vi "gui-demo.vi"() -> ()   [LabVIEW 2017]
uses:
  event-message-data.ctl
  list-commands-names.ctl
panel:
  in  "Array - String":string[](array[string])
  in  "create":bool
  in  "Instruction Tamplate":T1[](array[typedef])
  out "value":T2
  in  "stop":bool
  out "Instruction":string
  in  "initial preset":T3={"command-stack"=["label1:WAIT_SECONDS,2", "LIBX,demo-testflow.vi,WAIT", "JUMPCNT,label1,1", "FINISH"], "stack-config"=""}
  out "Instruction":string
  out "WAIT_SECONDS":T4
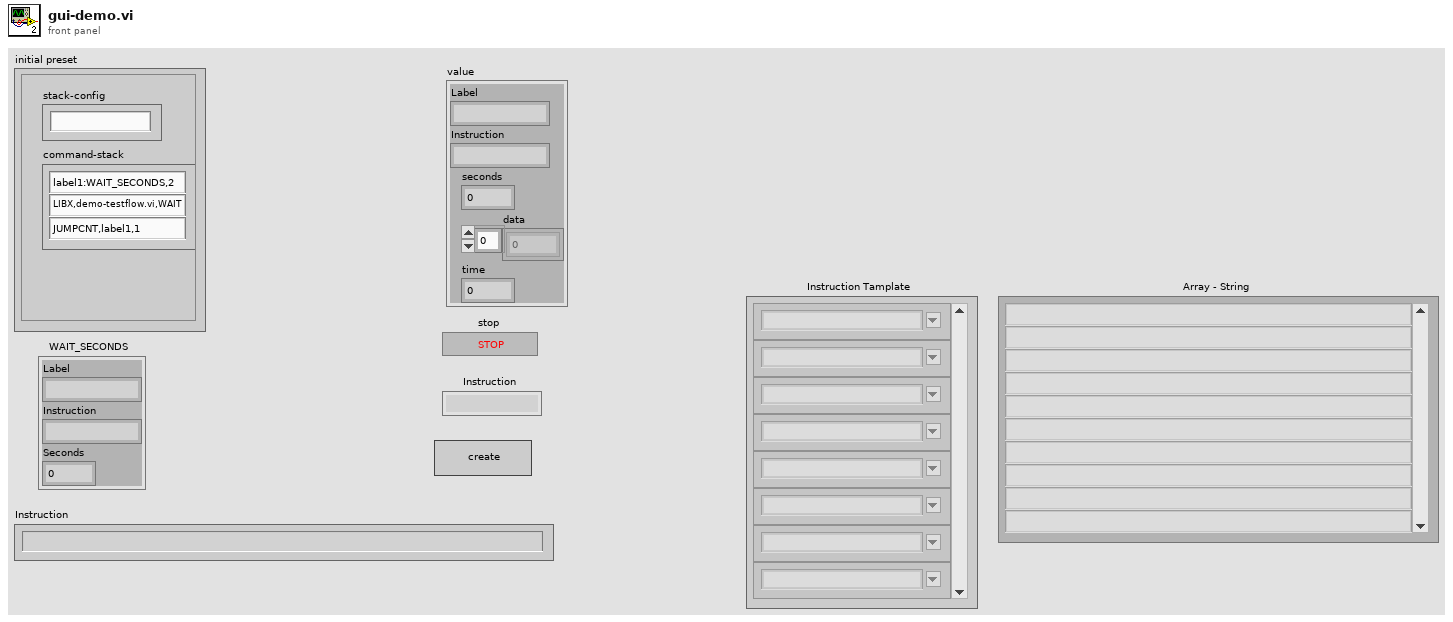
[diagram p1: front panel]
types:
  T1 = typedef "list-commands-names.ctl" = string
  T2 = cluster{"Label":string, "Instruction":string, "seconds":i32, "data":i32[], "time":i32}
  T3 = typedef "event-message-data.ctl" = cluster{"command-stack":string[], "stack-config":string}
  T4 = cluster{"Label":string, "Instruction":string, "Seconds":i32}
  T5 = cluster{"Label":string, "Instruction":string, "seconds":i32, "data":i32[]}
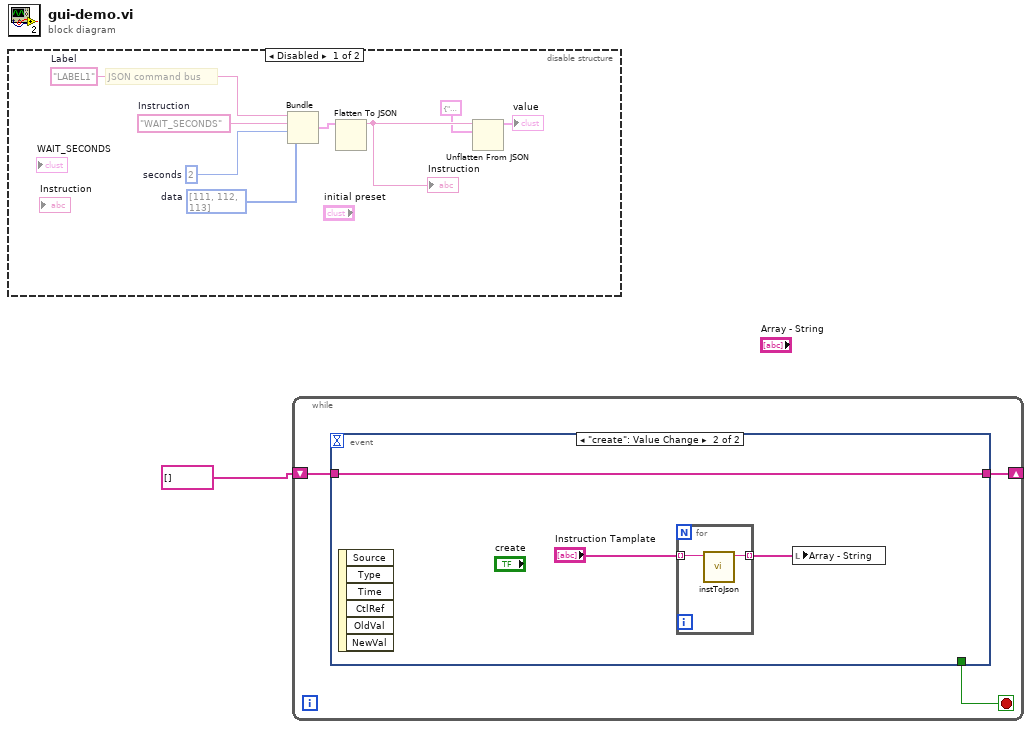
[diagram p0: block diagram]
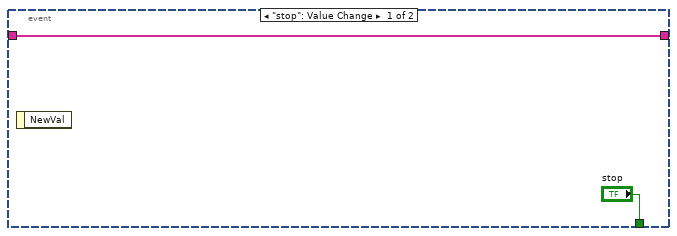
[diagram p3: hidden frame]
diagram:
  n1 = disable-structure shown="Disabled" {
    frame Disabled {
      w5 = i32[] [111, 112, 113]  # data
      w9 = "LABEL1"  # Label
      w8 = "WAIT_SECONDS"  # Instruction
      w6 = 2  # seconds
      # "JSON command bus"
      n2 = Bundle("Label"=w9, "Instruction"=w8, "seconds"=w6, "data"=w5) -> (w7:T5)  [unwired: 1 in]
      n3 = Flatten To JSON(anything=w7) -> (JSON string=w4:string)  [unwired: 2 in, 1 out]
      "Instruction" <- w4
      n4 = Unflatten From JSON(JSON string=w4, type and defaults=T2 {"Label"="", "Instruction"="", "seconds"=0, "data"=[], "time"=0} ("output cluster")) -> (value=→"value":T2)  [unwired: 5 in, 1 out]
    }
    frame Enabled {
    }
  }
  n5 = while {
    shift-right: [w11] -> _
    shift-left: string[] [] -> [w10]
    stop <- w12 stop-if-true
    n6 = event shown="[1] \"create\": Value Change" {
      selector: _ -> [_ _]
      dyn-events: _ -> [_ _]
      timeout: _ -> [_ _]
      tunnel: ["stop" _] -> w12
      tunnel: [w13 w17] -> w11
      tunnel: w10 -> [w13 w17]
      event "stop": Value Change {
        n7 = event-data() -> ()  [unwired: 1 in, 1 out]
      }
      event "create": Value Change {
        n8 = event-data() -> ()  [unwired: 1 in, 6 out]
        n9 = for {
          tunnel: [w19] -> w15 mode=indexing
          tunnel: "Instruction Tamplate" -> [w18] mode=indexing
          n10 = call "instToJson.vi"("instruction type"=w18) -> ("instruction template"=w19:string)  [unwired: 10 in]
        }
        n11 = local write "Array - String"(w15) -> ()
      }
    }
  }
